vi "IND560 Determine Units.vi"(8 "Error In":errorcluster, 11 "read buffer":string) -> (0 "Error Out":errorcluster, 3 "String":string)   [LabVIEW 2016]
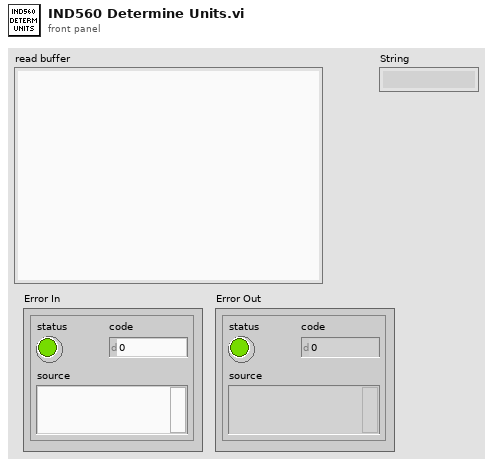
[diagram p1: front panel]
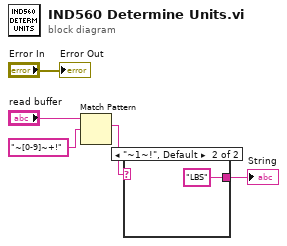
[diagram p0: block diagram]
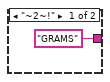
[diagram p2: hidden frame]
diagram:
  n1 = Match Pattern(string="read buffer", regular expression="~[0-9]~+!") -> (match substring=w3:string)  [unwired: 1 in, 3 out]
  n2 = case shown="\"~1~!\", Default" w3 {
    tunnel: ["GRAMS" "LBS"] -> w4
    frame "~2~!" {
    }
    frame "~1~!", Default {
    }
  }
  "String" <- w4
  "Error Out" <- "Error In"
